vi "16-ParseLengthTypeID.vi"(11 "BITS in in":bool[](array[boolean])) -> (2 "Length Type ID":T1(ring), 3 "BITS out":bool[](array[boolean]))   [LabVIEW 2019, in "16.lvlib"]
uses:
  16.lvlib
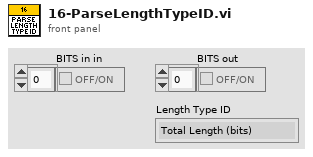
[diagram p1: front panel]
types:
  T1 = enum8{"Total Length (bits)", "Number of Subpackets"}
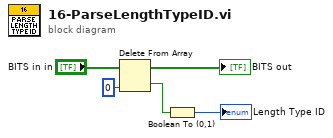
[diagram p0: block diagram]
diagram:
  n1 = Delete From Array(array="BITS in in", index=0) -> (deleted portion=w5:bool, array with subset deleted=→"BITS out":bool[])  [unwired: 1 in]
  n2 = Boolean To (0,1)(Boolean=w5) -> (0, 1=→"Length Type ID":i16)
